vi "Get Wirable Objects from Selection.vi"(8 "error in (no error)":errorcluster, 11 "SelList[]":refnum<vi>[](array[refnum])) -> (0 "error out":errorcluster, 1 "Parsed Selection List (Geographic Rows)":cluster{"Selection List":T2[]}[](array[cluster]), 2 "Controls, Constants, and Source Tunnels":T1[](array[typedef]), 3 "Indicators and Sink Tunnels":T1[](array[typedef]))   [LabVIEW 2016]
uses:
  <resource>/dialog/QuickDrop/plugins/_WireMultipleSupport/Node Terminal Info.ctl
  <resource>/dialog/QuickDrop/plugins/_WireMultipleSupport/Available Non-Node.ctl
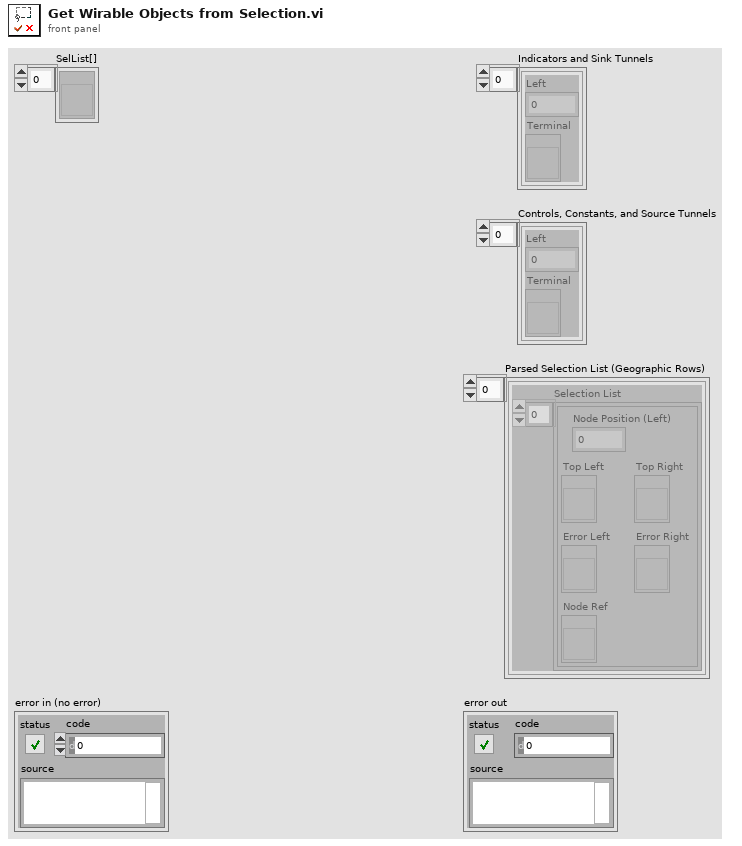
[diagram p1: front panel]
types:
  T1 = typedef "Available Non-Node.ctl" = cluster{"Left":i32, "Terminal":refnum<vi>}
  T2 = typedef "Node Terminal Info.ctl" = cluster{"Node Position (Left)":i32, "Node Ref":refnum<vi>, "Top Left":refnum<vi>, "Top Right":refnum<vi>, "Error Left":refnum<vi>, "Error Right":refnum<vi>}
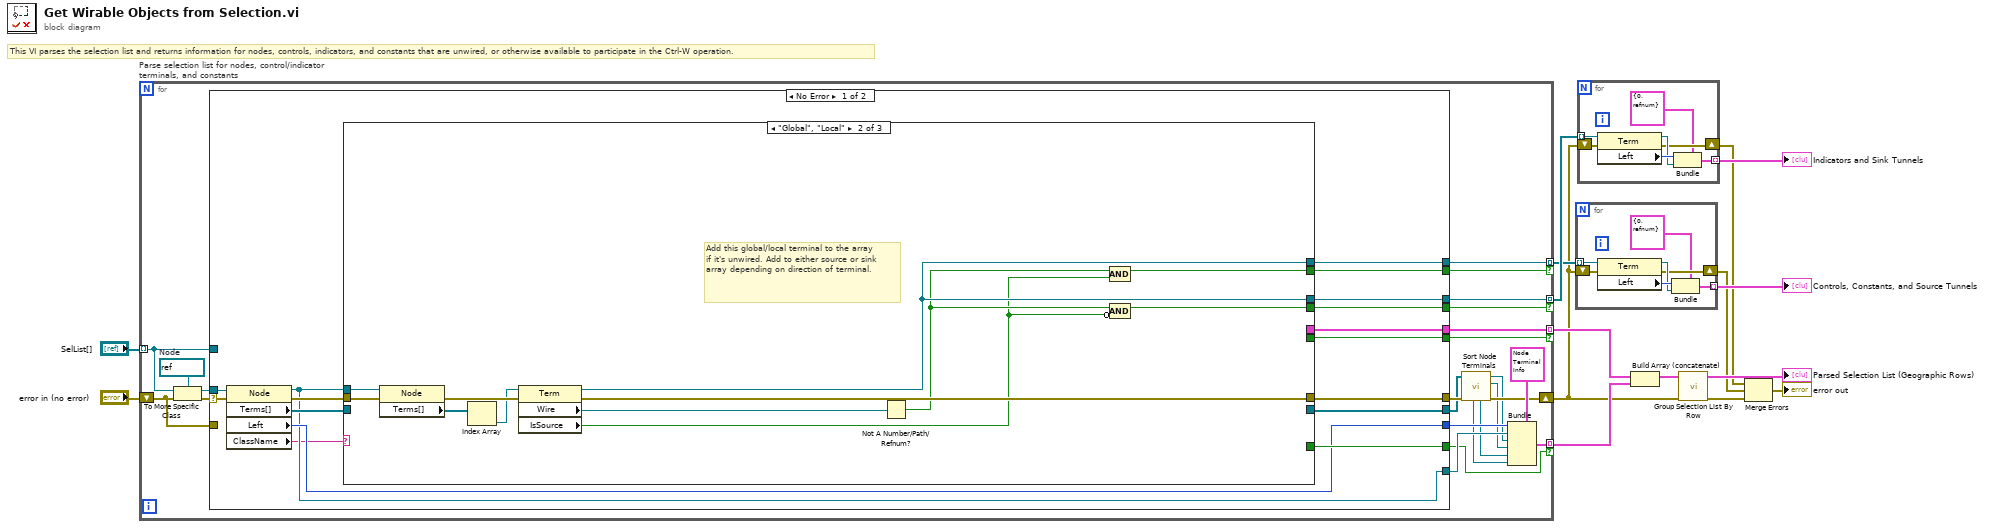
[diagram p0: block diagram]
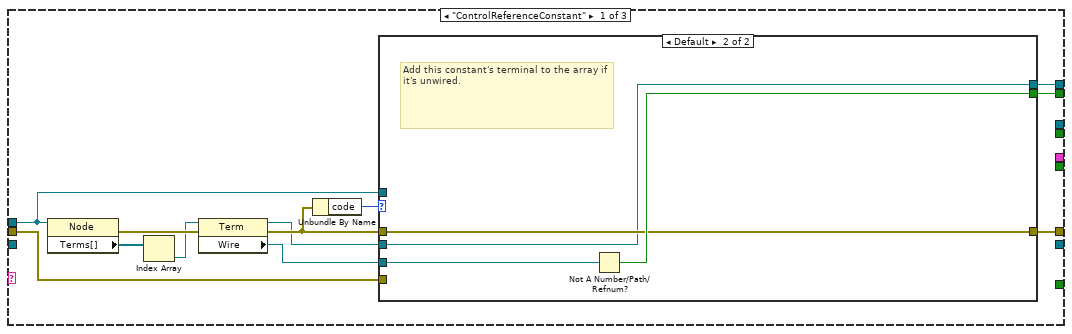
[diagram p2: hidden frame]
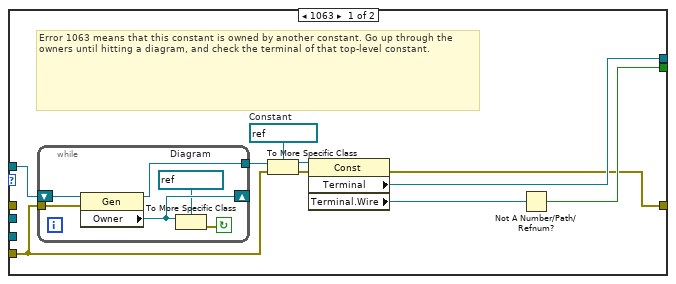
[diagram p3: hidden frame]
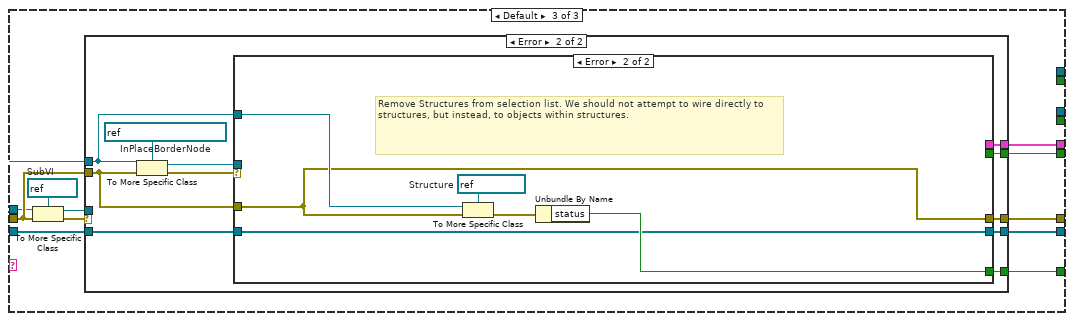
[diagram p4: hidden frame]
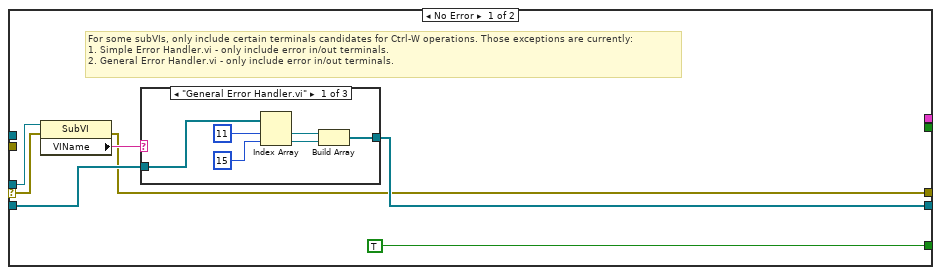
[diagram p5: hidden frame]
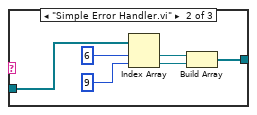
[diagram p6: hidden frame]
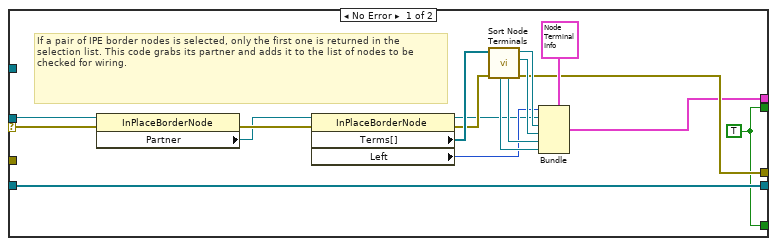
[diagram p8: hidden frame]
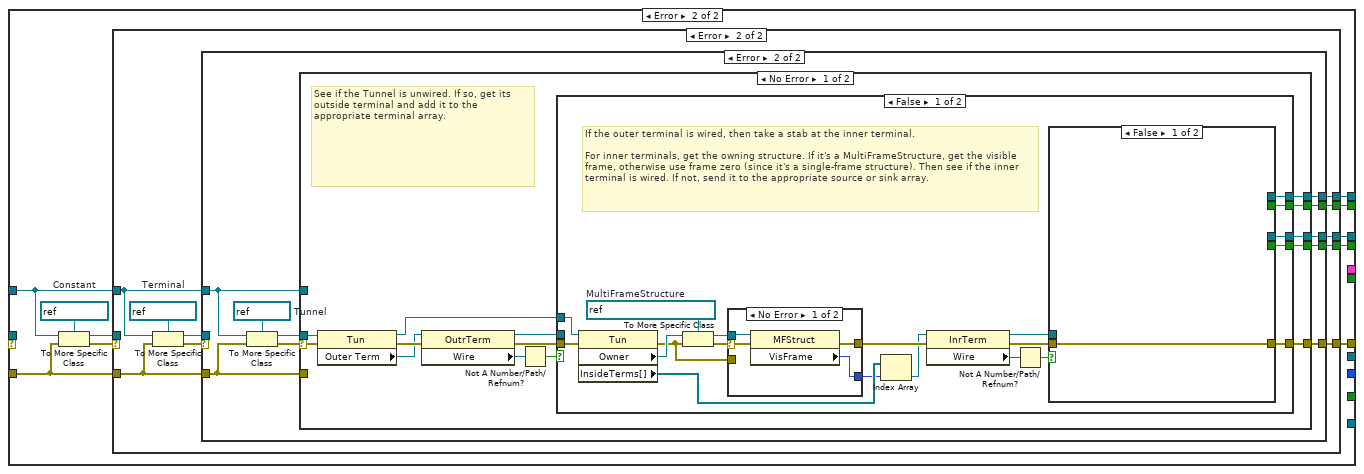
[diagram p9: hidden frame]
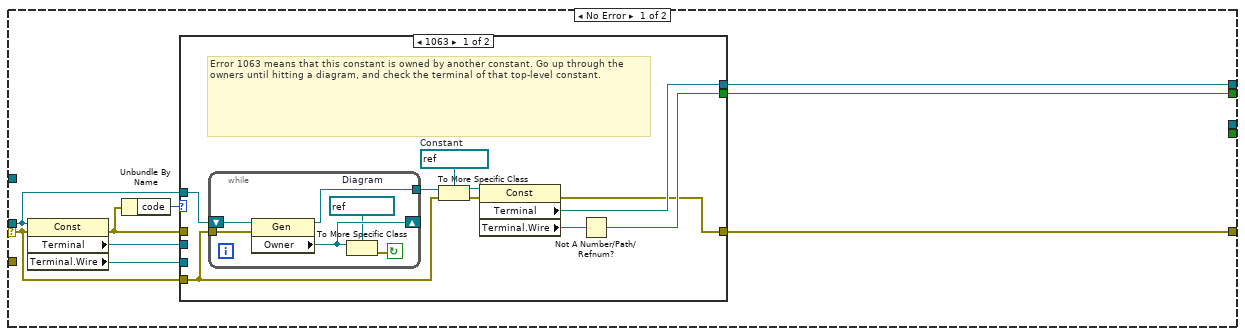
[diagram p10: hidden frame]
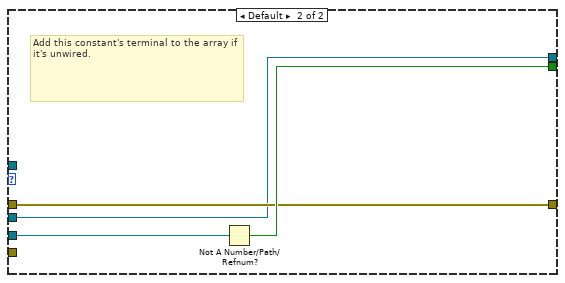
[diagram p11: hidden frame]
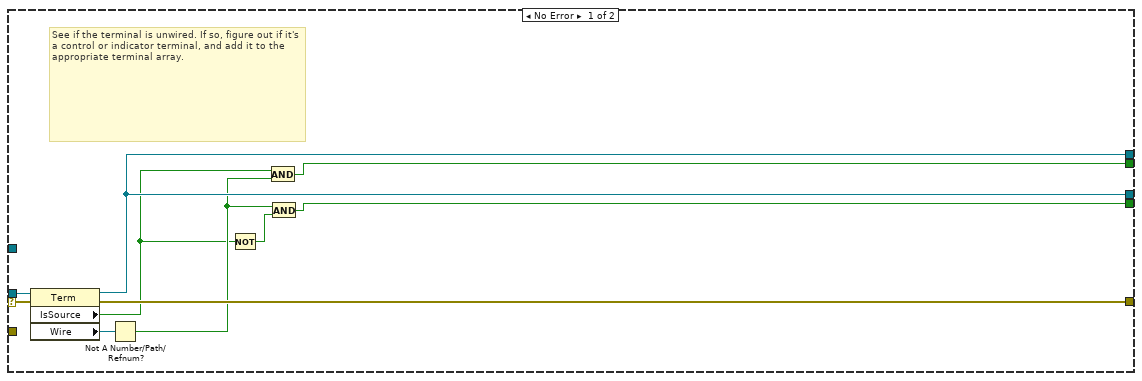
[diagram p12: hidden frame]
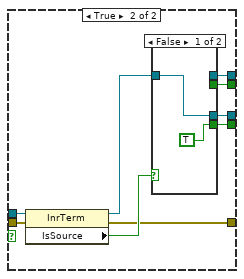
[diagram p13: hidden frame]
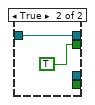
[diagram p14: hidden frame]
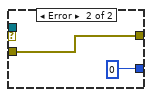
[diagram p15: hidden frame]
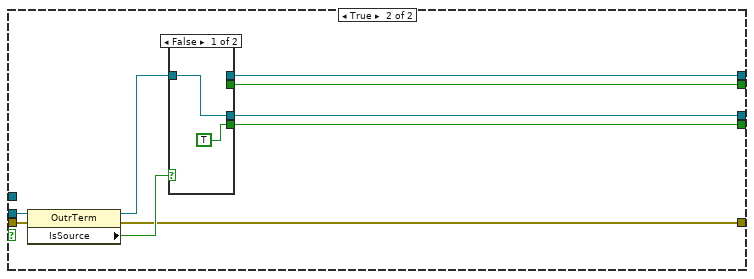
[diagram p16: hidden frame]
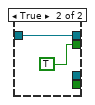
[diagram p17: hidden frame]
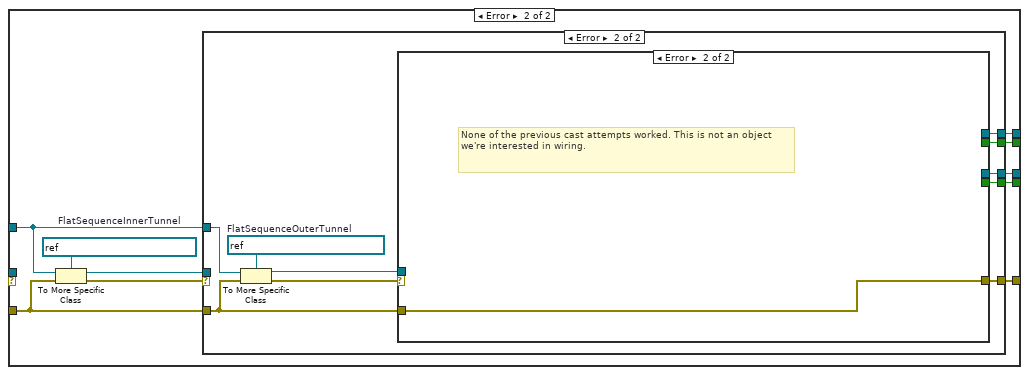
[diagram p18: hidden frame]
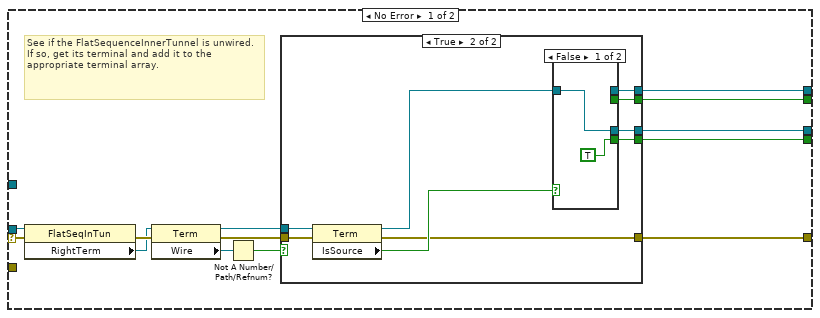
[diagram p19: hidden frame]
diagram:
  # "This VI parses the selection list and returns information for nodes, controls, indicators, and constants that are unwired, or otherwise available to participate in the Ctrl-W operation."
  n1 = for "Parse selection list for nodes, control/indicator terminals, and constants" {
    shift-right: [w26] -> w4
    shift-left: "error in (no error)" -> [w36]
    tunnel: "SelList[]" -> [w19] mode=indexing
    tunnel: [w34] -> w12 mode=indexing if=w16
    tunnel: [w33] -> w6 mode=indexing if=w32
    tunnel: [w31] -> w7 mode=indexing if=w30
    tunnel: [w18] -> w15 mode=indexing if=w17
    w20 = refnum<vi> refnum  # Node
    n2 = To More Specific Class(target class=w20, reference=w19, error in=w36) -> (specific class reference=w38:refnum<vi>, error out=w37:errorcluster)
    n3 = case shown="No Error" w37 {
      selector: w37 -> [w54 _]
      tunnel: w38 -> [w53 _]
      tunnel: [w49 _] -> w25
      tunnel: [w50 w170] -> w27
      tunnel: w36 -> [_ w171]
      tunnel: w19 -> [_ w169]
      tunnel: [w47 _] -> w35
      tunnel: [w48 _] -> w16
      tunnel: [w42 w168] -> w33
      tunnel: [w41 w167] -> w32
      tunnel: [w40 w166] -> w31
      tunnel: [w39 w165] -> w30
      tunnel: [w44 _] -> w28
      tunnel: [w46 _] -> w18
      tunnel: [w45 _] -> w17
      frame No Error {
        n4 = property class="Node"(reference=w53, error in=w54) -> (reference out=w44:refnum<vi>, error out=w51:errorcluster, "Terms[]"=w52:refnum<vi>[], "Left"=w47:i32, "ClassName"=w43:string)
        n5 = case shown="\"Global\", \"Local\"" w43 {
          tunnel: w52 -> [_ _ w109]
          tunnel: w51 -> [w64 w92 w105]
          tunnel: [w62 w96 w104] -> w50
          tunnel: [_ _ w103] -> w49
          tunnel: [_ _ w102] -> w48
          tunnel: [_ _ w101] -> w46
          tunnel: [_ _ w100] -> w45
          tunnel: w44 -> [w63 w97 w99]
          tunnel: [w61 w91 _] -> w42
          tunnel: [w60 w89 _] -> w41
          tunnel: [_ w91 _] -> w40
          tunnel: [_ w88 _] -> w39
          frame "ControlReferenceConstant" {
            n6 = property class="Node"(reference=w63) -> (error out=w65:errorcluster, "Terms[]"=w59:refnum<vi>[])  [unwired: 1 in, 1 out]
            n7 = Index Array(array=w59) -> (element=w56:refnum<vi>)  [unwired: 1 in]
            n8 = property class="Term"(reference=w56, error in=w65) -> (reference out=w55:refnum<vi>, error out=w58:errorcluster, "Wire"=w57:refnum<vi>)
            n9 = Unbundle By Name(w58) -> ("code"=w66:i32)
            n10 = case shown="Default" w66 {
              tunnel: w57 -> [_ w86]
              tunnel: [w73 w85] -> w60
              tunnel: w58 -> [_ w84]
              tunnel: [w68 w84] -> w62
              tunnel: w55 -> [_ w83]
              tunnel: [w69 w83] -> w61
              tunnel: w64 -> [w67 _]
              tunnel: w63 -> [w76 _]
              frame 1063 {
                w74 = refnum<vi> refnum  # Constant
                # "Error 1063 means that this constant is owned by another constant. Go up through the owners until hitting a diagram, and check the terminal of that top-level constant."
                n11 = while {
                  tunnel: w67 -> [w82]
                  shift-right: [w80] -> _
                  shift-left: w76 -> [w81]
                  tunnel: [w77] -> w75
                  stop <- w78 continue-if-true
                  w79 = refnum<vi> refnum  # Diagram
                  n12 = property class="Gen"(reference=w81, error in=w82) -> (reference out=w77:refnum<vi>, "Owner"=w80:refnum<vi>)  [unwired: 1 out]
                  n13 = To More Specific Class(target class=w79, reference=w80) -> (error out=w78:errorcluster)  [unwired: 1 in, 1 out]
                }
                n14 = To More Specific Class(target class=w74, reference=w75, error in=w67) -> (specific class reference=w72:refnum<vi>, error out=w71:errorcluster)
                n15 = property class="Const"(reference=w72, error in=w71) -> (error out=w68:errorcluster, "Terminal"=w69:refnum<vi>, "Terminal.Wire"=w70:refnum<vi>)  [unwired: 1 out]
                n16 = Not A Number/Path/Refnum?(number/path/refnum=w70) -> (NaN/Path/Refnum?=w73:bool)
              }
              frame Default {
                # "Add this constant's terminal to the array if it's unwired."
                n17 = Not A Number/Path/Refnum?(number/path/refnum=w86) -> (NaN/Path/Refnum?=w85:bool)
              }
            }
          }
          frame "Global", "Local" {
            # "Add this global/local terminal to the array if it's unwired. Add to either source or sink array depending on direction of terminal."
            n18 = property class="Node"(reference=w97, error in=w92) -> (error out=w98:errorcluster, "Terms[]"=w95:refnum<vi>[])  [unwired: 1 out]
            n19 = Index Array(array=w95) -> (element=w93:refnum<vi>)  [unwired: 1 in]
            n20 = property class="Term"(reference=w93, error in=w98) -> (reference out=w91:refnum<vi>, error out=w96:errorcluster, "Wire"=w94:refnum<vi>, "IsSource"=w87:bool)
            n21 = Not A Number/Path/Refnum?(number/path/refnum=w94) -> (NaN/Path/Refnum?=w90:bool)
            n22 = Compound Arithmetic op=AND(w90, w87) -> (w89:bool)
            n23 = Compound Arithmetic op=AND(w90, invert w87) -> (w88:bool)
          }
          frame Default {
            w108 = refnum<vi> refnum  # SubVI
            n24 = To More Specific Class(target class=w108, reference=w99, error in=w105) -> (specific class reference=w106:refnum<vi>, error out=w107:errorcluster)
            n25 = case shown="Error" w107 {
              selector: w107 -> [w115 _]
              tunnel: w109 -> [w113 w133]
              tunnel: w106 -> [w116 _]
              tunnel: w105 -> [_ w135]
              tunnel: [w111 w134] -> w104
              tunnel: [w112 w132] -> w103
              tunnel: [TRUE w140] -> w102
              tunnel: w99 -> [_ w136]
              tunnel: [_ w131] -> w101
              tunnel: [_ w130] -> w100
              frame No Error {
                # "For some subVIs, only include certain terminals candidates for Ctrl-W operations. Those exceptions are currently:\n1. Simple Error Handler.vi - only include error in/out terminals.\n2. General Error Handler.vi - only include error in/out terminals."
                n26 = property class="SubVI"(reference=w116, error in=w115) -> (error out=w111:errorcluster, "VIName"=w114:string)  [unwired: 1 out]
                n27 = case shown="\"General Error Handler.vi\"" w114 {
                  tunnel: w113 -> [w122 w128 w129]
                  tunnel: [w119 w125 w129] -> w112
                  frame "General Error Handler.vi" {
                    n28 = Index Array(array=w122, index #1=11, index #2=15) -> (element #1=w121:refnum<vi>, element #2=w120:refnum<vi>)
                    n29 = Build Array(w121, w120) -> (w119:refnum<vi>[])
                  }
                  frame "Simple Error Handler.vi" {
                    n30 = Index Array(array=w128, index #1=6, index #2=9) -> (element #1=w127:refnum<vi>, element #2=w126:refnum<vi>)
                    n31 = Build Array(w127, w126) -> (w125:refnum<vi>[])
                  }
                  frame Default {
                  }
                }
              }
              frame Error {
                w138 = refnum<vi> refnum  # InPlaceBorderNode
                n32 = To More Specific Class(target class=w138, reference=w136, error in=w135) -> (specific class reference=w139:refnum<vi>, error out=w137:errorcluster)
                n33 = case shown="Error" w137 {
                  selector: w137 -> [w151 _]
                  tunnel: [w141 w161] -> w140
                  tunnel: w139 -> [w142 _]
                  tunnel: w136 -> [_ w160]
                  tunnel: w135 -> [_ w159]
                  tunnel: [w145 w159] -> w134
                  tunnel: w133 -> [w157 w158]
                  tunnel: [w157 w158] -> w132
                  tunnel: [w143 _] -> w131
                  tunnel: [w141 _] -> w130
                  frame No Error {
                    w141 = TRUE
                    # "If a pair of IPE border nodes is selected, only the first one is returned in the selection list. This code grabs its partner and adds it to the list of nodes to be checked for wiring."
                    n34 = property class="InPlaceBorderNode"(reference=w142, error in=w151) -> (error out=w150:errorcluster, "Partner"=w149:refnum<vi>)  [unwired: 1 out]
                    n35 = property class="InPlaceBorderNode"(reference=w149, error in=w150) -> (reference out=w144:refnum<vi>, error out=w146:errorcluster, "Terms[]"=w147:refnum<vi>[], "Left"=w148:i32)
                    n36 = call <resource>:"Sort Node Terminals.vi"("error in (no error)"=w146, "Terms in"=w147) -> ("error out"=w145:errorcluster, "Top Right"=w154:refnum<vi>, "Top Left"=w153:refnum<vi>, "Error Left"=w155:refnum<vi>, "Error Right"=w156:refnum<vi>)  [unwired: 5 in]
                    n37 = Bundle(cluster=T2 {"Node Position (Left)"=0, "Node Ref"=refnum, "Top Left"=refnum, "Top Right"=refnum, "Error Left"=refnum, "Error Right"=refnum}, "Node Position (Left)"=w148, "Node Ref"=w144, "Top Left"=w153, "Top Right"=w154, "Error Left"=w155, "Error Right"=w156) -> (w143:T2)
                  }
                  frame Error {
                    w163 = refnum<vi> refnum  # Structure
                    # "Remove Structures from selection list. We should not attempt to wire directly to structures, but instead, to objects within structures."
                    n38 = To More Specific Class(target class=w163, reference=w160, error in=w159) -> (error out=w162:errorcluster)  [unwired: 1 out]
                    n39 = Unbundle By Name(w162) -> ("status"=w161:bool)
                  }
                }
              }
            }
          }
        }
      }
      frame Error {
        w164 = refnum<vi> refnum  # Constant
        n40 = To More Specific Class(target class=w164, reference=w169, error in=w171) -> (specific class reference=w172:refnum<vi>, error out=w173:errorcluster)
        n41 = case shown="Error" w173 {
          selector: w173 -> [w176 _]
          tunnel: w171 -> [_ w209]
          tunnel: w172 -> [w174 _]
          tunnel: [w180 w210] -> w170
          tunnel: w169 -> [_ w208]
          tunnel: [w177 w207] -> w168
          tunnel: [w181 w205] -> w167
          tunnel: [_ w206] -> w166
          tunnel: [_ w204] -> w165
          frame No Error {
            n42 = property class="Const"(reference=w174, error in=w176) -> (error out=w175:errorcluster, "Terminal"=w178:refnum<vi>, "Terminal.Wire"=w182:refnum<vi>)  [unwired: 1 out]
            n43 = Unbundle By Name(w175) -> ("code"=w179:i32)
            n44 = case shown="1063" w179 {
              tunnel: w182 -> [_ w202]
              tunnel: [w189 w201] -> w181
              tunnel: w175 -> [_ w200]
              tunnel: [w184 w200] -> w180
              tunnel: w178 -> [_ w199]
              tunnel: [w185 w199] -> w177
              tunnel: w176 -> [w183 _]
              tunnel: w174 -> [w192 _]
              frame 1063 {
                w190 = refnum<vi> refnum  # Constant
                # "Error 1063 means that this constant is owned by another constant. Go up through the owners until hitting a diagram, and check the terminal of that top-level constant."
                n45 = while {
                  tunnel: w183 -> [w198]
                  shift-right: [w196] -> _
                  shift-left: w192 -> [w197]
                  tunnel: [w193] -> w191
                  stop <- w194 continue-if-true
                  w195 = refnum<vi> refnum  # Diagram
                  n46 = property class="Gen"(reference=w197, error in=w198) -> (reference out=w193:refnum<vi>, "Owner"=w196:refnum<vi>)  [unwired: 1 out]
                  n47 = To More Specific Class(target class=w195, reference=w196) -> (error out=w194:errorcluster)  [unwired: 1 in, 1 out]
                }
                n48 = To More Specific Class(target class=w190, reference=w191, error in=w183) -> (specific class reference=w188:refnum<vi>, error out=w187:errorcluster)
                n49 = property class="Const"(reference=w188, error in=w187) -> (error out=w184:errorcluster, "Terminal"=w185:refnum<vi>, "Terminal.Wire"=w186:refnum<vi>)  [unwired: 1 out]
                n50 = Not A Number/Path/Refnum?(number/path/refnum=w186) -> (NaN/Path/Refnum?=w189:bool)
              }
              frame Default {
                # "Add this constant's terminal to the array if it's unwired."
                n51 = Not A Number/Path/Refnum?(number/path/refnum=w202) -> (NaN/Path/Refnum?=w201:bool)
              }
            }
          }
          frame Error {
            w203 = refnum<vi> refnum  # Terminal
            n52 = To More Specific Class(target class=w203, reference=w208, error in=w209) -> (specific class reference=w211:refnum<vi>, error out=w212:errorcluster)
            n53 = case shown="Error" w212 {
              selector: w212 -> [w222 _]
              tunnel: w211 -> [w220 _]
              tunnel: [w221 w230] -> w210
              tunnel: w209 -> [_ w229]
              tunnel: w208 -> [_ w223]
              tunnel: [w218 w227] -> w207
              tunnel: [w218 w225] -> w206
              tunnel: [w217 w226] -> w205
              tunnel: [w216 w224] -> w204
              frame No Error {
                # "See if the terminal is unwired. If so, figure out if it's a control or indicator terminal, and add it to the appropriate terminal array."
                n54 = property class="Term"(reference=w220, error in=w222) -> (reference out=w218:refnum<vi>, error out=w221:errorcluster, "IsSource"=w214:bool, "Wire"=w219:refnum<vi>)
                n55 = Not A Number/Path/Refnum?(number/path/refnum=w219) -> (NaN/Path/Refnum?=w215:bool)
                n56 = Not(x=w214) -> (.not. x?=w213:bool)
                n57 = And(x=w214, y=w215) -> (x .and. y?=w217:bool)
                n58 = And(x=w215, y=w213) -> (x .and. y?=w216:bool)
              }
              frame Error {
                w232 = refnum<vi> refnum  # Tunnel
                n59 = To More Specific Class(target class=w232, reference=w223, error in=w229) -> (specific class reference=w228:refnum<vi>, error out=w231:errorcluster)
                n60 = case shown="No Error" w231 {
                  selector: w231 -> [w246 _]
                  tunnel: [w239 w304] -> w230
                  tunnel: w229 -> [_ w306]
                  tunnel: w228 -> [w245 _]
                  tunnel: [w237 w303] -> w227
                  tunnel: [w236 w302] -> w226
                  tunnel: [w235 w301] -> w225
                  tunnel: [w234 w300] -> w224
                  tunnel: w223 -> [_ w307]
                  frame No Error {
                    # "See if the Tunnel is unwired. If so, get its outside terminal and add it to the appropriate terminal array."
                    n61 = property class="Tun"(reference=w245, error in=w246) -> (reference out=w233:refnum<vi>, error out=w244:errorcluster, "Outer Term"=w243:refnum<vi>)
                    n62 = property class="OutrTerm"(reference=w243, error in=w244) -> (reference out=w238:refnum<vi>, error out=w240:errorcluster, "Wire"=w242:refnum<vi>)
                    n63 = Not A Number/Path/Refnum?(number/path/refnum=w242) -> (NaN/Path/Refnum?=w241:bool)
                    n64 = case shown="False" w241 {
                      tunnel: w240 -> [w266 w294]
                      tunnel: [w256 w292] -> w239
                      tunnel: w238 -> [_ w295]
                      tunnel: [w255 w291] -> w237
                      tunnel: [w254 w289] -> w236
                      tunnel: [w253 w288] -> w235
                      tunnel: [w252 w287] -> w234
                      tunnel: w233 -> [w265 _]
                      frame False {
                        w263 = refnum<vi> refnum  # MultiFrameStructure
                        # "If the outer terminal is wired, then take a stab at the inner terminal.\n\nFor inner terminals, get the owning structure. If it's a MultiFrameStructure, get the visible frame, otherwise use frame zero (since it's a single-frame structure). Then see if the inner terminal is wired. If not, send it to the appropriate source or sink array."
                        n65 = property class="Tun"(reference=w265, error in=w266) -> (error out=w260:errorcluster, "Owner"=w264:refnum<vi>, "InsideTerms[]"=w259:refnum<vi>[])  [unwired: 1 out]
                        n66 = To More Specific Class(target class=w263, reference=w264, error in=w260) -> (specific class reference=w261:refnum<vi>, error out=w262:errorcluster)
                        n67 = case shown="No Error" w262 {
                          selector: w262 -> [w284 _]
                          tunnel: w261 -> [w283 _]
                          tunnel: [w282 w286] -> w257
                          tunnel: [w281 u32 0] -> w258
                          tunnel: w260 -> [_ w286]
                          frame No Error {
                            n68 = property class="MFStruct"(reference=w283, error in=w284) -> (error out=w282:errorcluster, "VisFrame"=w281:u32)  [unwired: 1 out]
                          }
                          frame Error {
                          }
                        }
                        n69 = Index Array(array=w259, index=w258) -> (element=w250:refnum<vi>)
                        n70 = property class="InrTerm"(reference=w250, error in=w257) -> (reference out=w249:refnum<vi>, error out=w251:errorcluster, "Wire"=w248:refnum<vi>)
                        n71 = Not A Number/Path/Refnum?(number/path/refnum=w248) -> (NaN/Path/Refnum?=w247:bool)
                        n72 = case shown="False" w247 {
                          tunnel: [w267 w274] -> w256
                          tunnel: [_ w273] -> w255
                          tunnel: [_ w272] -> w254
                          tunnel: [_ w271] -> w253
                          tunnel: [_ w270] -> w252
                          tunnel: w251 -> [w267 w269]
                          tunnel: w249 -> [_ w268]
                          frame False {
                          }
                          frame True {
                            n73 = property class="InrTerm"(reference=w268, error in=w269) -> (reference out=w275:refnum<vi>, error out=w274:errorcluster, "IsSource"=w276:bool)
                            n74 = case shown="False" w276 {
                              tunnel: [_ w280] -> w273
                              tunnel: w275 -> [w278 w280]
                              tunnel: [_ TRUE] -> w272
                              tunnel: [w278 _] -> w271
                              tunnel: [TRUE _] -> w270
                              frame False {
                              }
                              frame True {
                              }
                            }
                          }
                        }
                      }
                      frame True {
                        n75 = property class="OutrTerm"(reference=w295, error in=w294) -> (reference out=w290:refnum<vi>, error out=w292:errorcluster, "IsSource"=w293:bool)
                        n76 = case shown="False" w293 {
                          tunnel: [_ w299] -> w291
                          tunnel: w290 -> [w297 w299]
                          tunnel: [_ TRUE] -> w289
                          tunnel: [w297 _] -> w288
                          tunnel: [TRUE _] -> w287
                          frame False {
                          }
                          frame True {
                          }
                        }
                      }
                    }
                  }
                  frame Error {
                    w309 = refnum<vi> refnum  # FlatSequenceInnerTunnel
                    n77 = To More Specific Class(target class=w309, reference=w307, error in=w306) -> (specific class reference=w305:refnum<vi>, error out=w308:errorcluster)
                    n78 = case shown="Error" w308 {
                      selector: w308 -> [w317 _]
                      tunnel: w307 -> [_ w346]
                      tunnel: w306 -> [_ w342]
                      tunnel: w305 -> [w316 _]
                      tunnel: [w315 w341] -> w304
                      tunnel: [w314 w340] -> w303
                      tunnel: [w313 w339] -> w302
                      tunnel: [w312 w338] -> w301
                      tunnel: [w311 w337] -> w300
                      frame No Error {
                        # "See if the FlatSequenceInnerTunnel is unwired. If so, get its terminal and add it to the appropriate terminal array."
                        n79 = property class="FlatSeqInTun"(reference=w316, error in=w317) -> (error out=w322:errorcluster, "RightTerm"=w310:refnum<vi>)  [unwired: 1 out]
                        n80 = property class="Term"(reference=w310, error in=w322) -> (reference out=w318:refnum<vi>, error out=w319:errorcluster, "Wire"=w321:refnum<vi>)
                        n81 = Not A Number/Path/Refnum?(number/path/refnum=w321) -> (NaN/Path/Refnum?=w320:bool)
                        n82 = case shown="True" w320 {
                          tunnel: w319 -> [w323 w331]
                          tunnel: [w323 w329] -> w315
                          tunnel: w318 -> [_ w332]
                          tunnel: [_ w328] -> w314
                          tunnel: [_ w326] -> w313
                          tunnel: [_ w325] -> w312
                          tunnel: [_ w324] -> w311
                          frame False {
                          }
                          frame True {
                            n83 = property class="Term"(reference=w332, error in=w331) -> (reference out=w327:refnum<vi>, error out=w329:errorcluster, "IsSource"=w330:bool)
                            n84 = case shown="False" w330 {
                              tunnel: [_ w336] -> w328
                              tunnel: w327 -> [w334 w336]
                              tunnel: [_ TRUE] -> w326
                              tunnel: [w334 _] -> w325
                              tunnel: [TRUE _] -> w324
                              frame False {
                              }
                              frame True {
                              }
                            }
                          }
                        }
                      }
                      frame Error {
                        w345 = refnum<vi> refnum  # FlatSequenceOuterTunnel
                        n85 = To More Specific Class(target class=w345, reference=w346, error in=w342) -> (specific class reference=w343:refnum<vi>, error out=w344:errorcluster)
                        n86 = case shown="Error" w344 {
                          selector: w344 -> [w352 _]
                          tunnel: w343 -> [w353 _]
                          tunnel: w342 -> [_ w374]
                          tunnel: [w351 w374] -> w341
                          tunnel: [w350 _] -> w340
                          tunnel: [w349 _] -> w339
                          tunnel: [w348 _] -> w338
                          tunnel: [w347 _] -> w337
                          frame No Error {
                            # "See if the FlatSequenceOuterTunnel is unwired. If so, get its terminal and add it to the appropriate terminal array."
                            n87 = property class="FlatSeqOutTun"(reference=w353, error in=w352) -> (error out=w359:errorcluster, "OuterTerminal"=w358:refnum<vi>)  [unwired: 1 out]
                            n88 = property class="Term"(reference=w358, error in=w359) -> (reference out=w354:refnum<vi>, error out=w355:errorcluster, "Wire"=w357:refnum<vi>)
                            n89 = Not A Number/Path/Refnum?(number/path/refnum=w357) -> (NaN/Path/Refnum?=w356:bool)
                            n90 = case shown="True" w356 {
                              tunnel: w355 -> [w360 w368]
                              tunnel: [w360 w366] -> w351
                              tunnel: w354 -> [_ w369]
                              tunnel: [_ w365] -> w350
                              tunnel: [_ w363] -> w349
                              tunnel: [_ w362] -> w348
                              tunnel: [_ w361] -> w347
                              frame False {
                              }
                              frame True {
                                n91 = property class="Term"(reference=w369, error in=w368) -> (reference out=w364:refnum<vi>, error out=w366:errorcluster, "IsSource"=w367:bool)
                                n92 = case shown="False" w367 {
                                tunnel: [_ w373] -> w365
                                tunnel: w364 -> [w371 w373]
                                tunnel: [_ TRUE] -> w363
                                tunnel: [w371 _] -> w362
                                tunnel: [TRUE _] -> w361
                                frame False {
                                }
                                frame True {
                                }
                                }
                              }
                            }
                          }
                          frame Error {
                            # "None of the previous cast attempts worked. This is not an object we're interested in wiring."
                          }
                        }
                      }
                    }
                  }
                }
              }
            }
          }
        }
      }
    }
    n93 = call <resource>:"Sort Node Terminals.vi"("error in (no error)"=w27, "Terms in"=w25) -> ("error out"=w26:errorcluster, "Top Right"=w23:refnum<vi>, "Top Left"=w24:refnum<vi>, "Error Left"=w22:refnum<vi>, "Error Right"=w21:refnum<vi>)  [unwired: 5 in]
    n94 = Bundle(cluster=T2 {"Node Position (Left)"=0, "Node Ref"=refnum, "Top Left"=refnum, "Top Right"=refnum, "Error Left"=refnum, "Error Right"=refnum}, "Node Position (Left)"=w35, "Node Ref"=w28, "Top Left"=w24, "Top Right"=w23, "Error Left"=w22, "Error Right"=w21) -> (w34:T2)
  }
  n95 = for {
    tunnel: w6 -> [w381] mode=indexing
    tunnel: [w378] -> w9 mode=indexing
    shift-right: [w376] -> w2
    shift-left: w4 -> [w377]
    n96 = property class="Term"(reference=w381, error in=w377) -> (reference out=w379:refnum<vi>, error out=w376:errorcluster, "Left"=w380:i32)
    n97 = Bundle(cluster=T1 {"Left"=0, "Terminal"=refnum} ("Available Non-Node"), "Left"=w380, "Terminal"=w379) -> (w378:T1)
  }
  "Controls, Constants, and Source Tunnels" <- w9
  n98 = for {
    tunnel: w7 -> [w388] mode=indexing
    tunnel: [w385] -> w8 mode=indexing
    shift-right: [w383] -> w1
    shift-left: w4 -> [w384]
    n99 = property class="Term"(reference=w388, error in=w384) -> (reference out=w386:refnum<vi>, error out=w383:errorcluster, "Left"=w387:i32)
    n100 = Bundle(cluster=T1 {"Left"=0, "Terminal"=refnum} ("Available Non-Node"), "Left"=w387, "Terminal"=w386) -> (w385:T1)
  }
  "Indicators and Sink Tunnels" <- w8
  n101 = Build Array (concatenate)(w15, w12) -> (w14:T2[])
  n102 = call <resource>:"Group Selection List By Row.vi"("error in (no error)"=w4, "Parsed Selection List"=w14) -> ("error out"=w11:errorcluster, "Parsed Selection List (Geographic Rows)"=→"Parsed Selection List (Geographic Rows)":cluster{"Selection List":T2[]}[])  [unwired: 8 in]
  n103 = Merge Errors(w1, w2, w11) -> (→"error out":errorcluster)
